vi "Parse Boarding Pass.vi"(11 "Boarding Pass":string) -> (1 "Seat ID":u32, 2 "Column":u32, 3 "Row":u32)   [LabVIEW 2020]
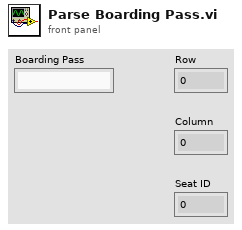
[diagram p1: front panel]
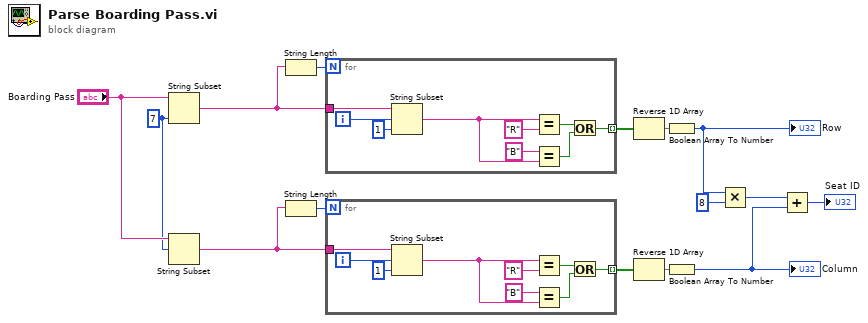
[diagram p0: block diagram]
diagram:
  w11 = 7 ("length (rest)")
  n1 = String Subset(string="Boarding Pass", length (rest)=w11) -> (substring=w10:string)  [unwired: 1 in]
  n2 = String Subset(string="Boarding Pass", offset (0)=w11) -> (substring=w6:string)  [unwired: 1 in]
  n3 = String Length(string=w10) -> (length=w13:i32)
  n4 = String Length(string=w6) -> (length=w9:i32)
  n5 = for {
    N: w13 -> [_]
    tunnel: w10 -> [w22]
    tunnel: [w16] -> w15 mode=indexing
    i -> [w21]
    n6 = String Subset(string=w22, offset (0)=w21, length (rest)=1 ("length (rest)")) -> (substring=w20:string)
    n7 = Equal?(x=w20, y="R") -> (x = y?=w18:bool)
    n8 = Equal?(x="B" ("y"), y=w20) -> (x = y?=w17:bool)
    n9 = Or(x=w18, y=w17) -> (x .or. y?=w16:bool)
  }
  n10 = for {
    N: w9 -> [_]
    tunnel: w6 -> [w31]
    tunnel: [w25] -> w7 mode=indexing
    i -> [w30]
    n11 = String Subset(string=w31, offset (0)=w30, length (rest)=1 ("length (rest)")) -> (substring=w29:string)
    n12 = Equal?(x=w29, y="R") -> (x = y?=w27:bool)
    n13 = Equal?(x="B" ("y"), y=w29) -> (x = y?=w26:bool)
    n14 = Or(x=w27, y=w26) -> (x .or. y?=w25:bool)
  }
  n15 = Reverse 1D Array(array=w15) -> (reversed array=w14:bool[])
  n16 = Reverse 1D Array(array=w7) -> (reversed array=w8:bool[])
  n17 = Boolean Array To Number(Boolean array=w14) -> (number=w5:u32)
  "Row" <- w5
  n18 = Boolean Array To Number(Boolean array=w8) -> (number=w2:u32)
  "Column" <- w2
  n19 = Multiply(x=w5, y=u32 8) -> (x*y=w3:u32)
  n20 = Add(x=w3, y=w2) -> (x+y=→"Seat ID":u32)
